vi "Ex6-polynomial curve fitting.vi"() -> ()   [LabVIEW 2021]
uses:
  <vilib>/httpClient/POSTBuffer.vi
  <vilib>/httpClient/LabVIEWHTTPClient.lvlib
panel:
  out "headers":string="HTTP/1.1 429 Too Many Requests\r\ndate: Mon, 02 Mar 2026 11:23:04 GMT\r\nserver: uvicorn\r\ncontent-length: 47\r\ncontent-type: application/json\r\n\r\n"
  out "body":string="{\"error\":\"Rate limit exceeded: 5 per 1 minute\"}"
  out "Cluster":cluster{"x":dbl[], "z":dbl[]}={"x"=[-50.0, -45.0, -40.0, -35.0, -30.0], "z"=[666.4828571428559, 479.1885714285711, 335.7371428571433, 236.12857142857195, 180.36285714285725]}
  out "XY Graph":cluster{"x":dbl[], "z":dbl[]}[](graph)=[{"x"=[-50.0, -45.0, -40.0, -35.0, -30.0], "z"=[670.1, 471.7, 336.5, 242.6, 177.0]}, {"x"=[-50.0, -45.0, -40.0, -35.0, -30.0], "z"=[666.4828571428559, 479.1885714285711, 335.7371428571433, 236.12857142857195, 180.36285714285725]}]
  in  "Data":cluster{"X":dbl[], "Y":dbl[], "Order":dbl}={"X"=[-50.0, -45.0, -40.0, -35.0, -30.0], "Y"=[670.1, 471.7, 336.5, 242.6, 177.0], "Order"=2.0}
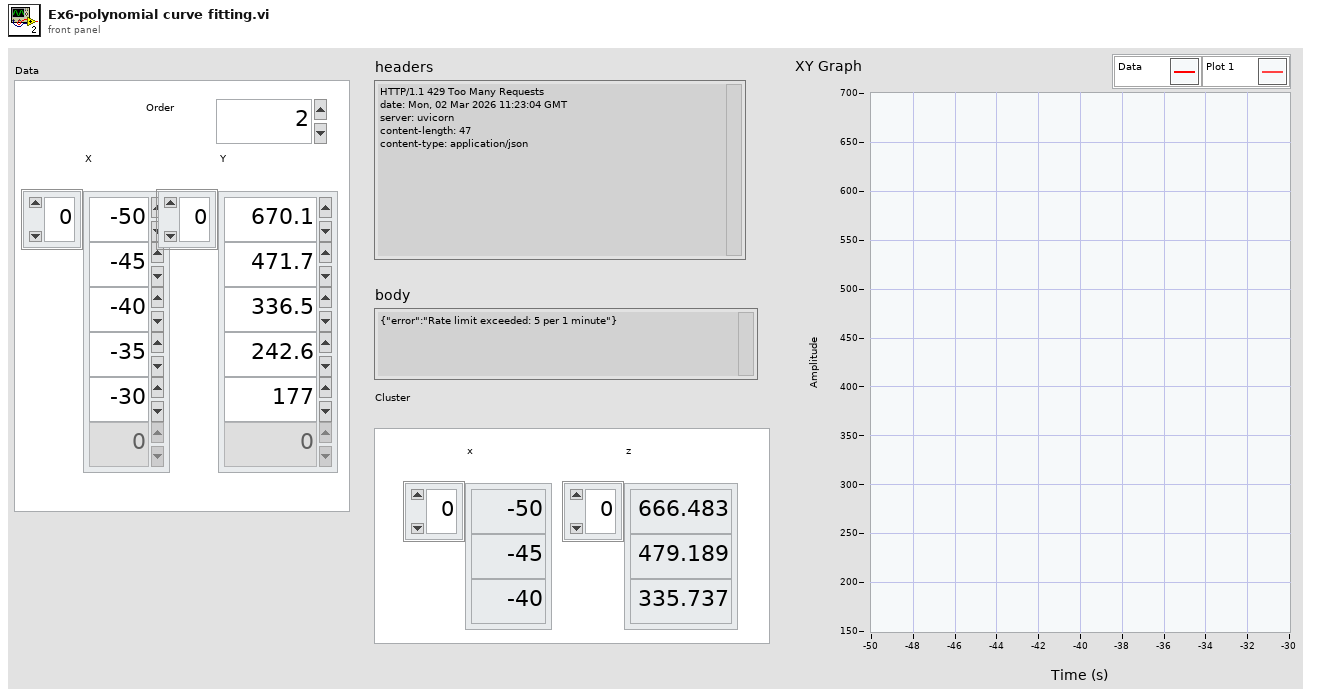
[diagram p1: front panel]
types:
  T1 = typedef "LabVIEWHTTPClient.lvlib/ClientHandle.ctl" = refnum<k1>
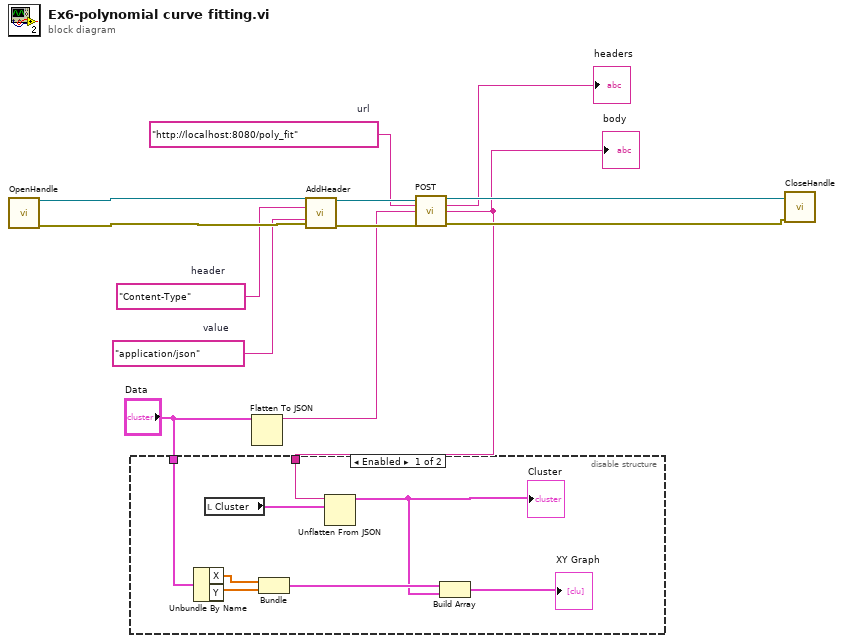
[diagram p0: block diagram]
diagram:
  w5 = "http://localhost:8080/poly_fit"  # url
  w8 = "application/json"  # value
  w9 = "Content-Type"  # header
  n1 = call <vilib>:"OpenHandle.vi"() -> ("client handle out"=w13:T1, "error out"=w12:errorcluster)  [unwired: 14 in]
  n2 = Flatten To JSON(anything="Data") -> (JSON string=w3:string)  [unwired: 2 in, 1 out]
  n3 = call <vilib>:"AddHeader.vi"("client handle"=w13, "header"=w9, "value"=w8, "error in (no error)"=w12) -> ("client handle out"=w7:T1, "error out"=w6:errorcluster)  [unwired: 10 in]
  n4 = call-poly <vilib>:"POST.vi"("client handle"=w7, "url"=w5, "buffer"=w3, "error in (no error)"=w6) -> ("client handle out"=w11:T1, "headers"=→"headers":string, "body"=w2:string, "error out"=w10:errorcluster)  [unwired: 8 in]
  "body" <- w2
  n5 = disable-structure shown="Enabled" {
    disable-tunnel: w2 -> [w20 _]
    disable-tunnel: "Data" -> [w19 _]
    frame Enabled {
      n6 = Unbundle By Name "Unbundle By Name"(w19) -> ("X"=w18:dbl[], "Y"=w17:dbl[])
      n7 = local read "Cluster"() -> (w21:cluster{"x":dbl[], "z":dbl[]})
      n8 = Bundle "Bundle"("X"=w18, "Y"=w17) -> (w16:cluster{"X":dbl[], "Y":dbl[]})  [unwired: 1 in]
      n9 = Unflatten From JSON(JSON string=w20, type and defaults=w21) -> (value=w15:cluster{"x":dbl[], "z":dbl[]})  [unwired: 5 in, 1 out]
      "Cluster" <- w15
      n10 = Build Array "Build Array"(w16, w15) -> (→"XY Graph":cluster{"x":dbl[], "z":dbl[]}[])
    }
    frame Disabled {
    }
  }
  n11 = call <vilib>:"CloseHandle.vi"("client handle"=w11, "error in (no error)"=w10) -> ()  [unwired: 13 in, 1 out]
